vi "S token.vi"(10 "regular expression":string, 11 "input string":string) -> (1 "after match":string, 2 "whole match":string, 3 "token found":bool)   [LabVIEW 2010]
uses:
  <vilib>/regexp/Match Regular Expression.xnode
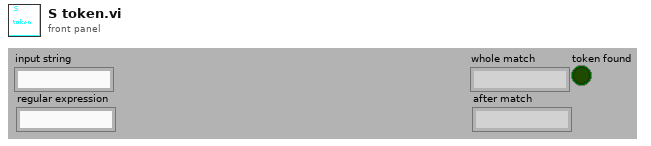
[diagram p1: front panel]
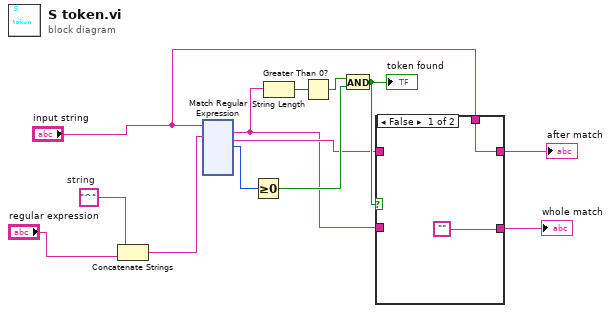
[diagram p0: block diagram]
diagram:
  w9 = "^"  # string
  n1 = Concatenate Strings(w9, "regular expression") -> (w7:string)
  n2 = xnode "Match Regular Expression"("input string"="input string", "regular expression"=w7) -> ("whole match"=w2:string, "after match"=w4:string, "offset past match"=w13:i32)  [unwired: 4 in, 4 out]
  n3 = Greater Or Equal To 0?(x=w13) -> (x >= 0?=w10:bool)
  n4 = String Length(string=w2) -> (length=w12:i32)
  n5 = Greater Than 0?(x=w12) -> (x > 0?=w11:bool)
  n6 = And(x=w11, y=w10) -> (x .and. y?=w6:bool)
  "token found" <- w6
  n7 = case shown="False" w6 {
    tunnel: [w15 w17] -> w5
    tunnel: w4 -> [_ w17]
    tunnel: ["" w16] -> w3
    tunnel: w2 -> [_ w16]
    tunnel: "input string" -> [w15 _]
    frame False {
    }
    frame True {
    }
  }
  "whole match" <- w3
  "after match" <- w5
